vi "search.vi"(6 "Small Cave Visited Twize":bool, 8 "Error In":errorcluster, 9 "Path(Nodes)":refnum<class "12_Cave.lvclass">[](array[class]), 10 "FronNode":refnum<class "12_Cave.lvclass">, 11 "NoOfPath":refnum<data-value>) -> (0 "Error Out":errorcluster, 1 "PathOut":refnum<class "12_Cave.lvclass">[](array[class]))   [LabVIEW 2020, in "2021_12.lvclass"]
uses:
  2021_12.lvclass
  12_Cave_class/12_Cave.lvclass
  475aab4c-7174-4909-b796-073f3a6cc18e.vi
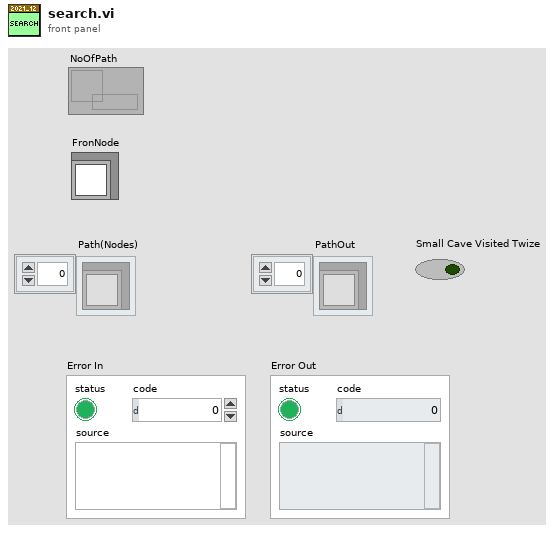
[diagram p1: front panel]
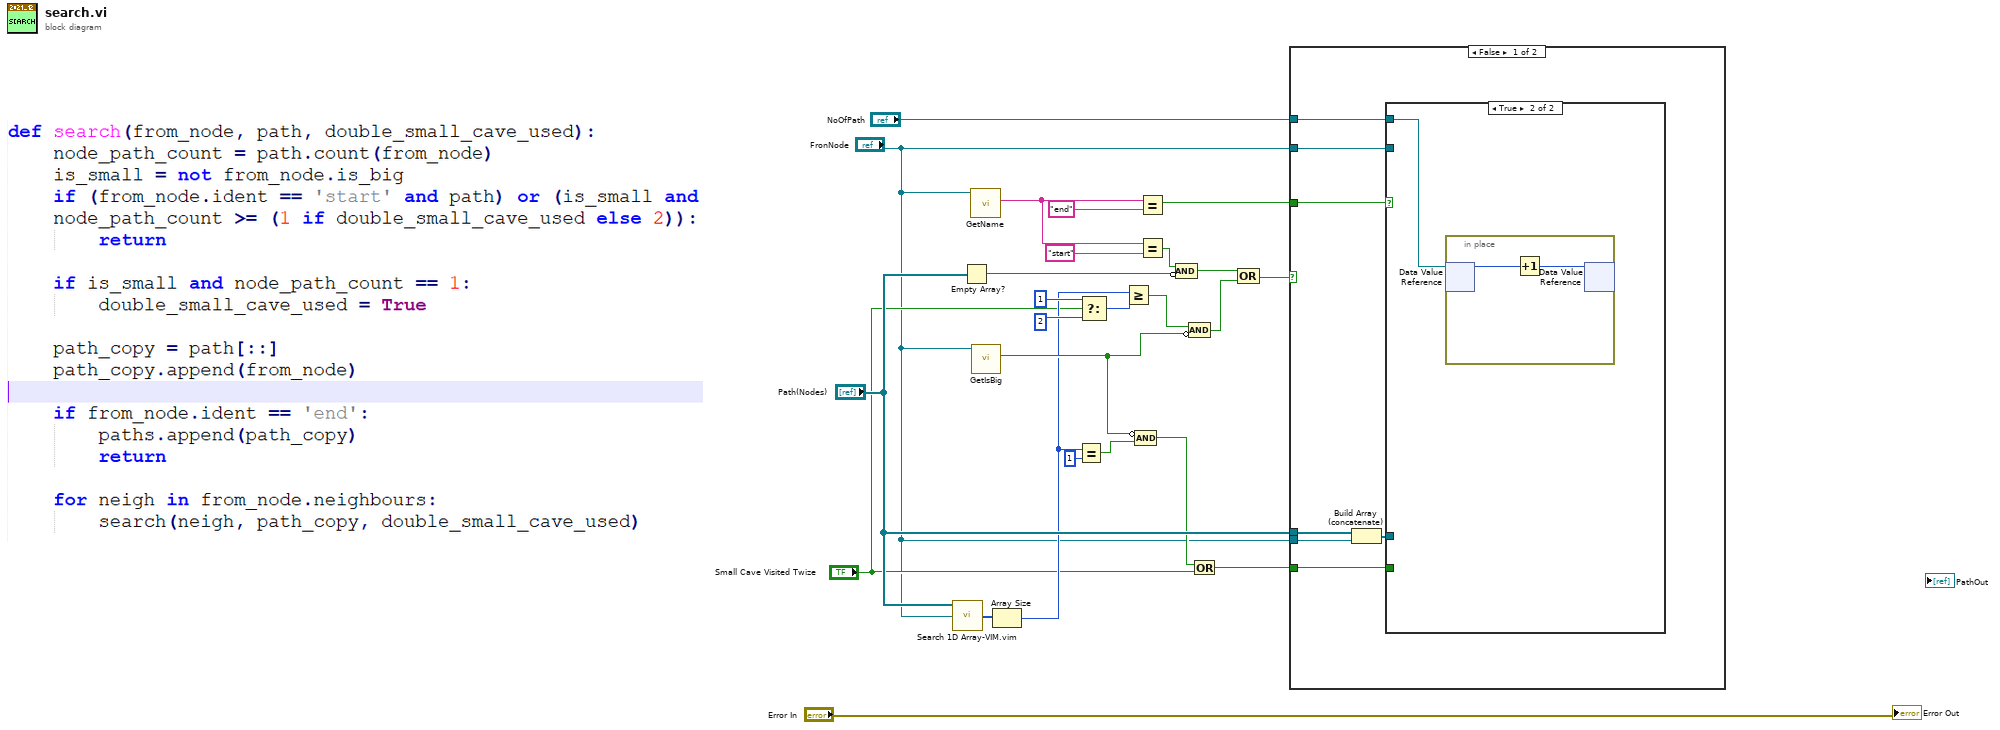
[diagram p0: block diagram]
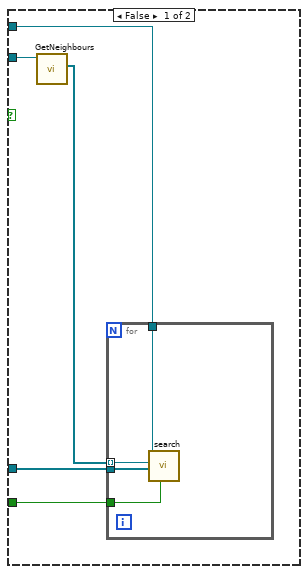
[diagram p2: hidden frame]
diagram:
  n1 = call "Search 1D Array-VIM.vim"("Array"="Path(Nodes)", "Element Data"="FronNode") -> ("Indices of Elements"=w22:i32[])  [unwired: 7 in]
  n2 = Empty Array?(array="Path(Nodes)") -> (empty?=w19:bool)
  n3 = call-dynamic "GetName.vi"("reference in"="FronNode") -> ("Name"=w20:string)  [unwired: 8 in, 2 out]
  n4 = call-dynamic "GetIsBig.vi"("reference in"="FronNode") -> ("Is Big"=w10:bool)  [unwired: 8 in, 2 out]
  n5 = Array Size(array=w22) -> (size(s)=w8:i32)
  n6 = Equal?(x=w8, y=1 ("t")) -> (x = y?=w6:bool)
  n7 = Select(t=1, s="Small Cave Visited Twize", f=2 ("t")) -> (s? t:f=w14:i32)
  n8 = Greater Or Equal?(x=w8, y=w14) -> (x >= y?=w15:bool)
  n9 = Compound Arithmetic op=AND(invert w10, w6) -> (w5:bool)
  n10 = Equal?(x=w20, y="end") -> (x = y?=w23:bool)
  n11 = Equal?(x=w20, y="start") -> (x = y?=w18:bool)
  n12 = Compound Arithmetic op=AND(w18, invert w19) -> (w17:bool)
  n13 = Compound Arithmetic op=AND(w15, invert w10) -> (w16:bool)
  n14 = Or(x=w5, y="Small Cave Visited Twize") -> (x .or. y?=w3:bool)
  n15 = Compound Arithmetic op=OR(w17, w16) -> (w11:bool)
  n16 = case shown="False" w11 {
    tunnel: w23 -> [w32 _]
    tunnel: "FronNode" -> [w31 _]
    tunnel: "Path(Nodes)" -> [w30 _]
    tunnel: w3 -> [w29 _]
    tunnel: "FronNode" -> [w28 _]
    tunnel: "NoOfPath" -> [w27 _]
    frame False {
      n17 = Build Array (concatenate)(w30, w31) -> (w26:refnum<class "12_Cave.lvclass">[])
      n18 = case shown="True" w32 {
        tunnel: w26 -> [w37 _]
        tunnel: w29 -> [w36 _]
        tunnel: w28 -> [w35 _]
        tunnel: w27 -> [w33 w42]
        frame False {
          n19 = call-dynamic "GetNeighbours.vi"("reference in"=w35) -> ("Neighbours"=w34:refnum<class "12_Cave.lvclass">[])  [unwired: 8 in, 2 out]
          n20 = for {
            tunnel: w37 -> [w41]
            tunnel: w34 -> [w40] mode=indexing
            tunnel: w36 -> [w39]
            tunnel: w33 -> [w38]
            n21 = call "search.vi"("Small Cave Visited Twize"=w39, "Path(Nodes)"=w41, "FronNode"=w40, "NoOfPath"=w38) -> ()  [unwired: 6 in, 2 out]
          }
        }
        frame True {
          n22 = in-place {
            n23 = in-place-dvr #1(w42) -> (w44:i32)  [unwired: 1 out]
            n24 = Increment(x=w44) -> (x+1=w43:i32)
            n25 = in-place-dvr #1(w43) -> ()  [unwired: 2 out]
          }
        }
      }
    }
    frame True {
    }
  }
  "Error Out" <- "Error In"
